vi "Add Items (inline).vi"(4 "indent":i32, 6 "Insertion index":i32, 8 "error in (no error)":errorcluster, 10 "Items to Add":refnum<class "BetterItem.lvclass">[](array[class]), 11 "BetterHandle in":refnum<class "BetterHandle.lvclass">) -> (0 "error out":errorcluster, 3 "BetterHandle out":refnum<class "BetterHandle.lvclass">)   [LabVIEW 2020, in "BetterDragAndDrop.lvlib" / "BetterHandle.lvclass"]
uses:
  BetterHandle.lvclass
  BetterTreeItem/BetterItem.lvclass
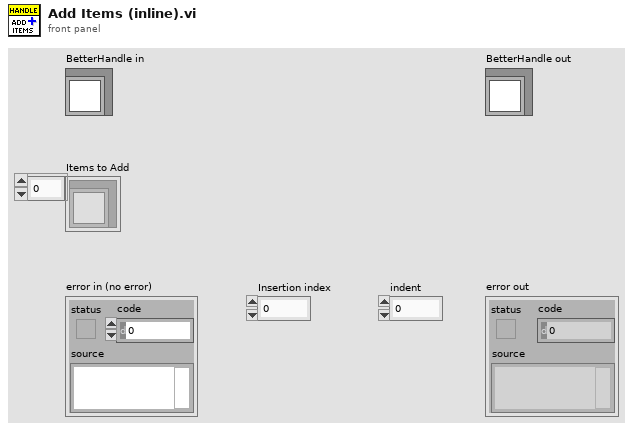
[diagram p1: front panel]
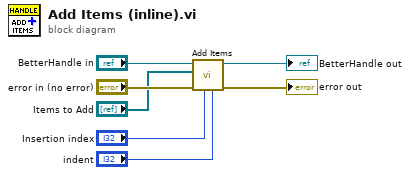
[diagram p0: block diagram]
diagram:
  n1 = call-dynamic "Add Items.vi"("indent"="indent", "Insertion index"="Insertion index", "error in (no error)"="error in (no error)", "Items to Add"="Items to Add", "BetterHandle in"="BetterHandle in") -> ("error out"=→"error out":errorcluster, "BetterHandle out"=→"BetterHandle out":refnum<class "BetterHandle.lvclass">)  [unwired: 5 in]
